vi "Integer Array.vi"   [LabVIEW 2020, in "Memory Manager Tests.lvlib" / "Malleable Type Tests.lvclass"]
uses:
  Malleable Type Tests.lvclass
  Malleable Type Tests.lvclass/Malleable Type Tests.ctl
  Source/Classes/Pointer/Pointer.lvclass
  b7fb4431-4503-4e6c-b996-b6c0db621e23.vi
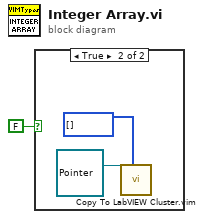
[diagram p0: block diagram]
diagram:
  n1 = case shown="True" FALSE {
    frame False {
    }
    frame True {
      n2 = call "Copy To LabVIEW Cluster.vim"("Type"=i32[] [], "Pointer in"=refnum<class "Pointer.lvclass"> refnum) -> ()  [unwired: 7 in, 3 out]
    }
  }
